vi "Keyboard4Shooter.vi"(6 "1D array":T1(array[ring])) -> (0 "Suction":bool, 1 "ShootOR(control)":bool, 2 "Shoot(control)":bool, 4 "Ejection":bool, 5 "AutoSearch":bool)   [LabVIEW 2011]
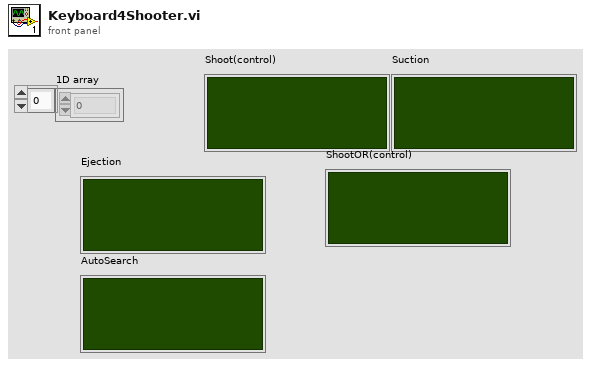
[diagram p1: front panel]
types:
  T1 = enum16{"0", "1", "2", "3", "4", "5", "6", "7", "8", "9", "A", "B", "C", "D", "E", "F", "G", "H", "I", "J", "K", "L", "M", "N", "O", "P", "Q", "R", "S", "T", "U", "V", "W", "X", "Y", "Z", "F1", "F2", "F3", "F4", "F5", "F6", "F7", "F8", "F9", "F10", "F11", "F12", "F13", "F14", "F15", "ADD", "BACK", "BACKSLASH", "CAPITAL", "COMMA", "DECIMAL", "DELETE", "DIVIDE", "DOWN", "END", "EQUALS", "ESCAPE", "GRAVE (`)", "HOME", "INSERT", "LBRACKET", "LCONTROL", "LEFT", "L ALT", "LSHIFT", "LWIN", "MINUS", "MULTIPLY", "NEXT", "NUMLOCK", "NUMPAD_0", "NUMPAD_1", "NUMPAD_2", "NUMPAD_3", "NUMPAD_4", "NUMPAD_5", "NUMPAD_6", "NUMPAD_7", "NUMPAD_8", "NUMPAD_9", "PAUSE", "PERIOD", "PRIOR (PG UP)", "RBRACKET", "RCONTROL", "RETURN", "RIGHT", "R ALT", "RSHIFT", "RWIN", "SCROLL", "SEMICOLON", "SLASH", "SPACE", "SUBTRACT", "TAB", "UP", "ENTER (num pad)", "' (quote)"}[]
  T2 = enum16{"0", "1", "2", "3", "4", "5", "6", "7", "8", "9", "A", "B", "C", "D", "E", "F", "G", "H", "I", "J", "K", "L", "M", "N", "O", "P", "Q", "R", "S", "T", "U", "V", "W", "X", "Y", "Z", "F1", "F2", "F3", "F4", "F5", "F6", "F7", "F8", "F9", "F10", "F11", "F12", "F13", "F14", "F15", "ADD", "BACK", "BACKSLASH", "CAPITAL", "COMMA", "DECIMAL", "DELETE", "DIVIDE", "DOWN", "END", "EQUALS", "ESCAPE", "GRAVE (`)", "HOME", "INSERT", "LBRACKET", "LCONTROL", "LEFT", "L ALT", "LSHIFT", "LWIN", "MINUS", "MULTIPLY", "NEXT", "NUMLOCK", "NUMPAD_0", "NUMPAD_1", "NUMPAD_2", "NUMPAD_3", "NUMPAD_4", "NUMPAD_5", "NUMPAD_6", "NUMPAD_7", "NUMPAD_8", "NUMPAD_9", "PAUSE", "PERIOD", "PRIOR (PG UP)", "RBRACKET", "RCONTROL", "RETURN", "RIGHT", "R ALT", "RSHIFT", "RWIN", "SCROLL", "SEMICOLON", "SLASH", "SPACE", "SUBTRACT", "TAB", "UP", "ENTER (num pad)", "' (quote)"}
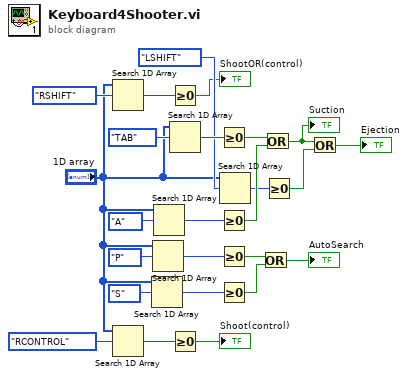
[diagram p0: block diagram]
diagram:
  n1 = Search 1D Array(1D array="1D array", element=T2."RSHIFT" ("keys pressed[0]")) -> (index of element=w22:i32)  [unwired: 1 in]
  n2 = Search 1D Array(1D array="1D array", element=T2."RCONTROL" ("keys pressed[0]")) -> (index of element=w25:i32)  [unwired: 1 in]
  n3 = Search 1D Array(1D array="1D array", element=T2."S" ("keys pressed[0]")) -> (index of element=w11:i32)  [unwired: 1 in]
  n4 = Search 1D Array(1D array="1D array", element=T2."P" ("keys pressed[0]")) -> (index of element=w8:i32)  [unwired: 1 in]
  n5 = Search 1D Array(1D array="1D array", element=T2."A" ("keys pressed[0]")) -> (index of element=w19:i32)  [unwired: 1 in]
  n6 = Greater Or Equal To 0?(x=w22) -> (x >= 0?=→"ShootOR(control)":bool)
  n7 = Search 1D Array(1D array="1D array", element=T2."TAB" ("keys pressed[0]")) -> (index of element=w16:i32)  [unwired: 1 in]
  n8 = Greater Or Equal To 0?(x=w25) -> (x >= 0?=→"Shoot(control)":bool)
  n9 = Greater Or Equal To 0?(x=w16) -> (x >= 0?=w20:bool)
  n10 = Greater Or Equal To 0?(x=w19) -> (x >= 0?=w21:bool)
  n11 = Greater Or Equal To 0?(x=w8) -> (x >= 0?=w12:bool)
  n12 = Greater Or Equal To 0?(x=w11) -> (x >= 0?=w13:bool)
  n13 = Search 1D Array(1D array="1D array", element=T2."LSHIFT" ("keys pressed[0]")) -> (index of element=w15:i32)  [unwired: 1 in]
  n14 = Or(x=w12, y=w13) -> (x .or. y?=→"AutoSearch":bool)
  n15 = Or(x=w20, y=w21) -> (x .or. y?=w2:bool)
  "Suction" <- w2
  n16 = Greater Or Equal To 0?(x=w15) -> (x >= 0?=w3:bool)
  n17 = Or(x=w2, y=w3) -> (x .or. y?=→"Ejection":bool)
